vi "Write to Protected Connection.vi"(8 "error in (no error)":errorcluster, 9 "Packet":refnum<class "IPacket.lvclass">, 10 "Connection Writer":refnum<class "ProtectedConnectionWriter.lvclass">, 11 "Write Strategy in":refnum<class "Write Strategy.lvclass">) -> (0 "error out":errorcluster)   [LabVIEW 2020, in "Network Messenger.lvlib" / "Write Strategy.lvclass"]
uses:
  <vilib>/gpm_packages/@cs/Network-interface/Source/Network Messenger/Write Strategy/Write Strategy.lvclass
  <vilib>/gpm_packages/@cs/Network-interface/Source/ProtectedConnectionWriter/ProtectedConnectionWriter.lvclass
  <vilib>/gpm_packages/@cs/Network-interface/Source/MessagingInterfaces/IPacket/IPacket.lvclass
  <vilib>/gpm_packages/@cs/Network-interface/Source/ProtectedConnectionWriter/ProtectedConnectionWriter.lvclass/ProtectedConnectionWriter.ctl
  <vilib>/gpm_packages/@cs/Network-interface/Source/Connection Reference/Connection Reference/Connection Reference.lvclass/Connection Reference.ctl
  <vilib>/gpm_packages/@cs/Network-interface/Source/Connection Reference/IConnection/IConnection.lvclass
  <vilib>/gpm_packages/@cs/Network-interface/Source/Network Messenger/Network Messenger.lvlib
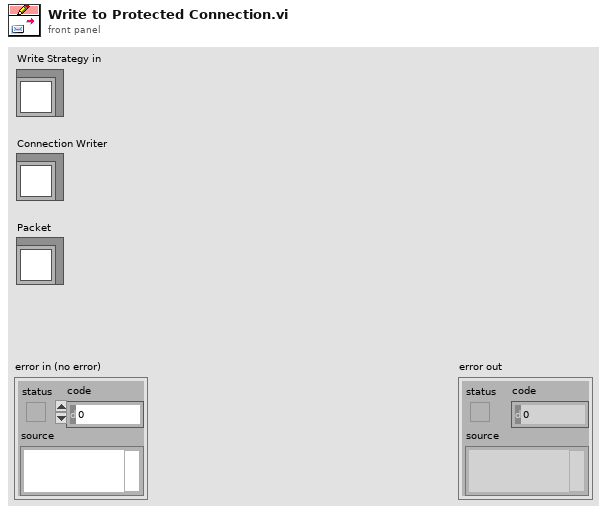
[diagram p1: front panel]
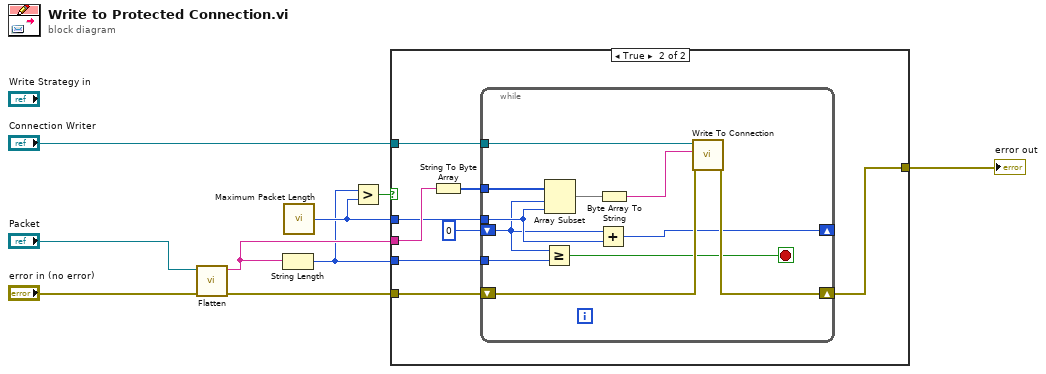
[diagram p0: block diagram]
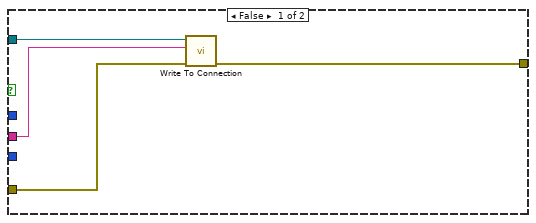
[diagram p2: hidden frame]
diagram:
  n1 = call-dynamic "Flatten.vi"("error in (no error)"="error in (no error)", "IPacket in"="Packet") -> ("error out"=w6:errorcluster, "Flattened Packet"=w4:string)  [unwired: 8 in]
  n2 = String Length(string=w4) -> (length=w1:i32)
  n3 = call <vilib>:"Maximum Packet Length.vi"() -> ("Max Packet Length"=w2:i32)
  n4 = Greater?(x=w1, y=w2) -> (0:w3:bool)
  n5 = case shown="True" w3 {
    tunnel: "Connection Writer" -> [w13 w21]
    tunnel: w6 -> [w12 w20]
    tunnel: [w11 w19] -> w5
    tunnel: w4 -> [w10 w18]
    tunnel: w2 -> [_ w17]
    tunnel: w1 -> [_ w14]
    frame False {
      n6 = call <vilib>:"Write To Connection.vi"("error in (no error)"=w12, "Data to Write"=w10, "ProtectedConnectionWriter in"=w13) -> ("error out"=w11:errorcluster)  [unwired: 8 in]
    }
    frame True {
      n7 = String To Byte Array(string=w18) -> (unsigned byte array=w16:u8[])
      n8 = while {
        tunnel: w21 -> [w32]
        shift-right: [w30] -> w19
        shift-left: w20 -> [w31]
        tunnel: w16 -> [w29]
        shift-right: [w26] -> _
        shift-left: 0 ("index") -> [w24]
        tunnel: w14 -> [w23]
        tunnel: w17 -> [w27]
        stop <- w22 stop-if-true
        n9 = Greater Or Equal?(x=w24, y=w23) -> (x >= y?=w22:bool)
        n10 = Array Subset(array=w29, index=w24, length=w27) -> (w25:u8[])
        n11 = Add(x=w24, y=w27) -> (x+y=w26:i32)
        n12 = Byte Array To String(unsigned byte array=w25) -> (string=w28:string)
        n13 = call <vilib>:"Write To Connection.vi"("error in (no error)"=w31, "Data to Write"=w28, "ProtectedConnectionWriter in"=w32) -> ("error out"=w30:errorcluster)  [unwired: 8 in]
      }
    }
  }
  "error out" <- w5
